vi "CRYSet Signal Type Dialog Front Panel.vi"(11 "Vi Ref":refnum<vi>) -> ()   [LabVIEW 2013]
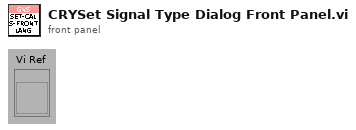
[diagram p1: front panel]
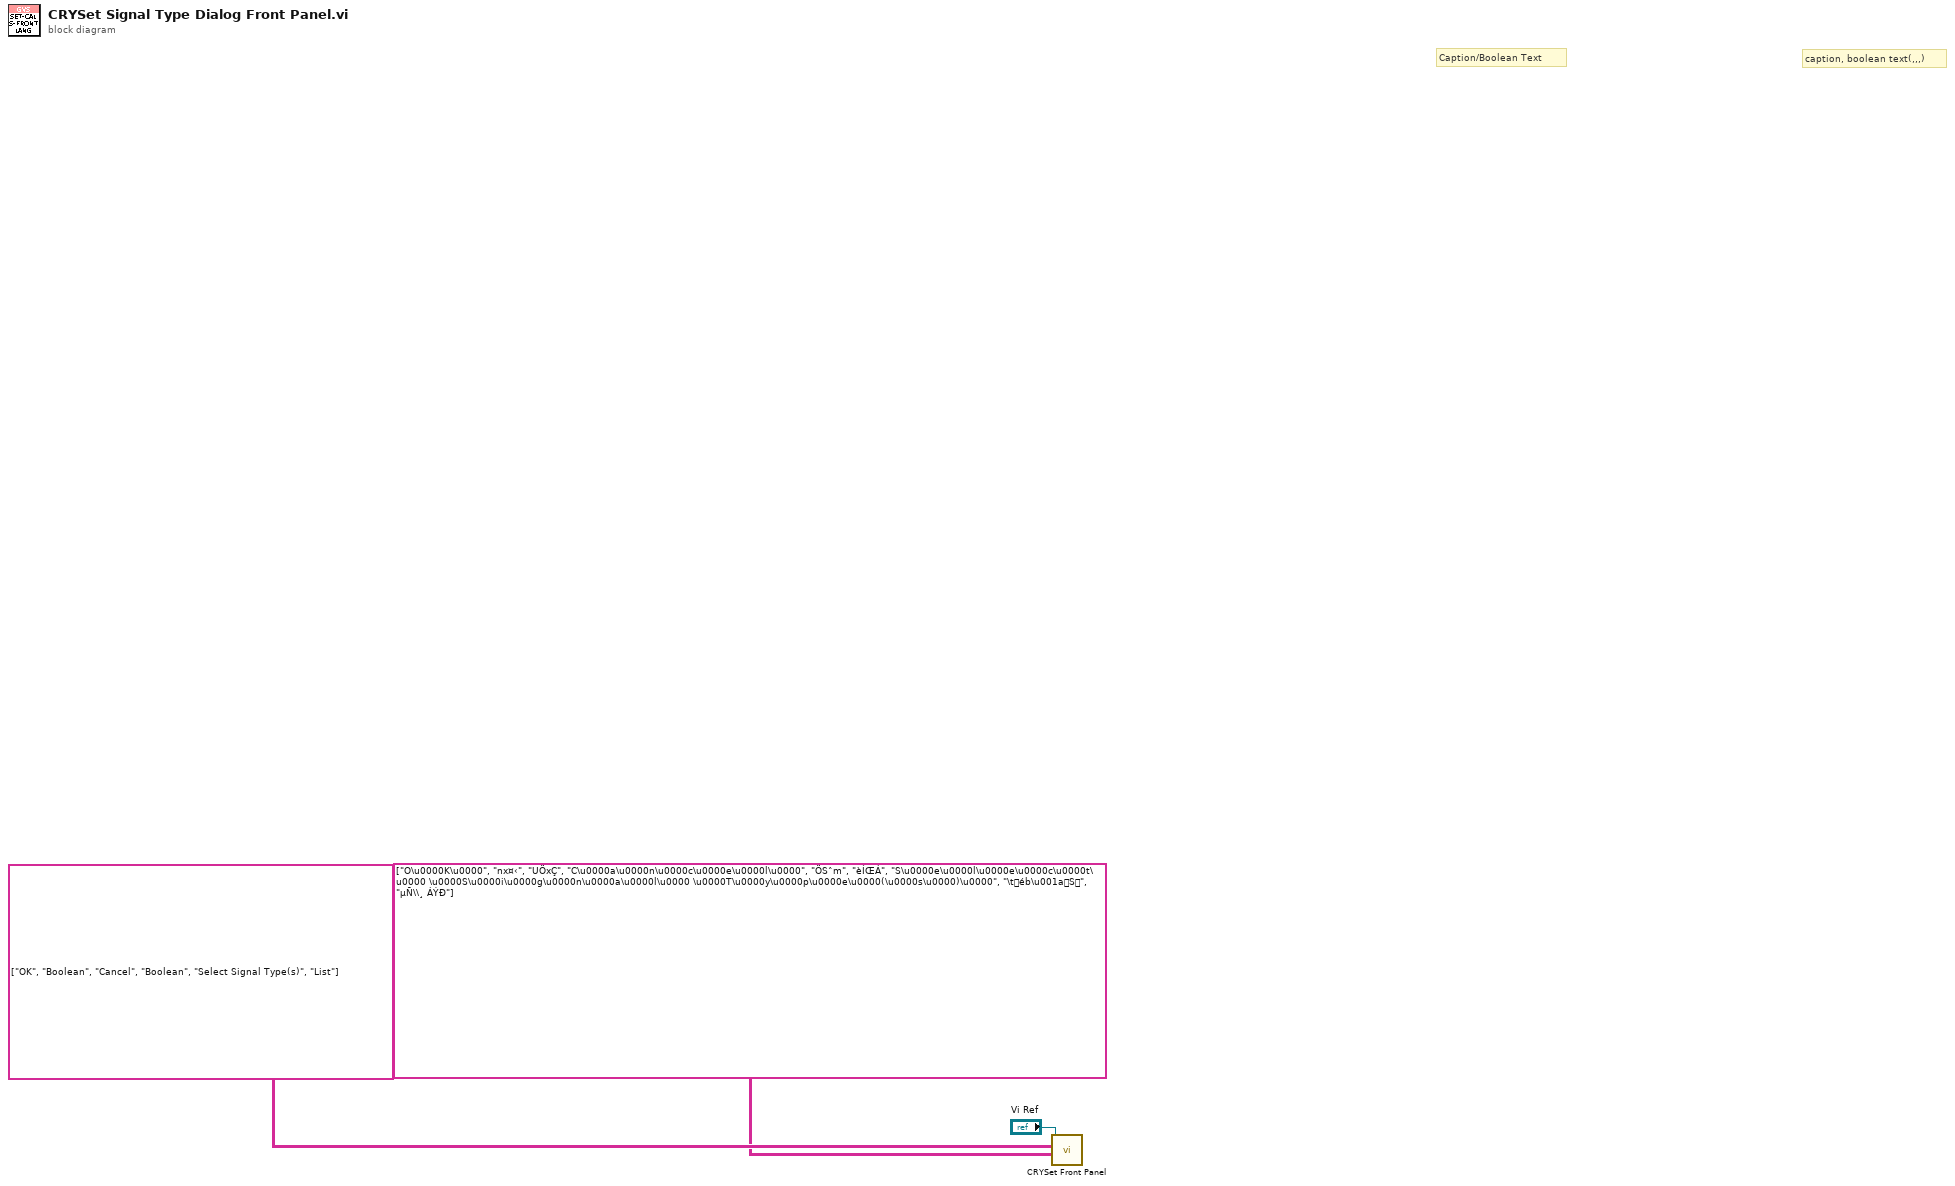
[diagram p0: block diagram]
diagram:
  # "caption, boolean text(,,,)"
  # "Caption/Boolean Text"
  n1 = call "CRYSet Front Panel.vi"("Caption(Boolean Text)"=string[][] [["O\u0000K\u0000", "nx¤‹", "UÖxÇ"], ["C\u0000a\u0000n\u0000c\u0000e\u0000l\u0000", "ÖSˆm", "èÍŒÁ"], ["S\u0000e\u0000l\u0000e\u0000c\u0000t\u0000 \u0000S\u0000i\u0000g\u0000n\u0000a\u0000l\u0000 \u0000T\u0000y\u0000p\u0000e\u0000(\u0000s\u0000)\u0000", "\téb\u001aS", "µÑ\\¸ ÁÝÐ"]], "Control ID and Type(Label Name, Type)"=string[][] [["OK", "Boolean"], ["Cancel", "Boolean"], ["Select Signal Type(s)", "List"]], "Vi Ref"="Vi Ref") -> ()  [unwired: 9 in]
